vi "系统设置.vi"() -> ()   [LabVIEW 2016]
uses:
  <vilib>/Utility/miscctls.llb/LVPointTypeDef.ctl
  <vilib>/ptbypt/NI_PtbyPt.lvlib
  <vilib>/Utility/config.llb/NI_LVConfig.lvlib
  PLC/PLC.lvlib
panel:
  in  "模块启用配置":bool
  in  "短信报警设置":bool
  in  "首页显示设置":bool
  in  "跨度核查":bool
  in  "空白核查":bool
  out "选项卡控件":enum32{"自由设定", "国标协议", "流量设定"}(tab)
  in  "24H周期设置":bool[](xcontrol)
  in  "运行间隔":i16=4 min=1 max=24
  in  "流量阈值":dbl=4.0 min=1.0 max=24.0
  in  "时间阈值":u16=4 min=1 max=24
  in  "周期设置":enum16{"自由设定", "国标协议", "流量设定"}(ring)
  out "x = y?":bool
  in  "质控启动日期":string(combo)="关闭"
  in  "跨度核查时间":u16(ring)=6 items=["00H", "01H", "02H", "03H", "04H", "05H", "06H", "07H", "08H", "09H", "10H", "11H", "12H", "13H", "14H", "15H", "16H", "17H", "18H", "19H", "20H", "21H", "22H", "23H", "关闭"]
  in  "空白核查时间":u16(ring)=2 items=["00H", "01H", "02H", "03H", "04H", "05H", "06H", "07H", "08H", "09H", "10H", "11H", "12H", "13H", "14H", "15H", "16H", "17H", "18H", "19H", "20H", "21H", "22H", "23H", "关闭"]
  in  "CODCr":bool
  in  "总磷总氮":bool
  in  "氨氮":bool
  in  "CODmn":bool
  in  "多参数":bool
  in  "输入密码":dbl
  in  "布尔":bool
  in  "副屏显示设置":bool
  in  "开机启动":bool caption="氨氮禁用"
  in  "运行模式":enum16{"维护模式", "常规模式", "应急模式", "质控模式"}(ring)
  # "注：周期设置分为自由设定和国标协议两种。\n1：选择自由设定情况下：运行间隔将不可选用并变灰色，周期设置可自由手动勾选\n2：选择国标协议情况下：周期时间将由运行间隔选择的时间决定，下方周期设置被禁用并无法手动勾选。\n3：选择流量设定情况下：瞬时流量连续超过流量阈值到达时间阈值设定值，仪器将自动开启测量。"
  # "自动运行启动参数"
  # "质控频次："
  # "空白核查时间："
  # "跨度核查时间："
  # "启动周期设置"
  # "m3/S"
  # "秒"
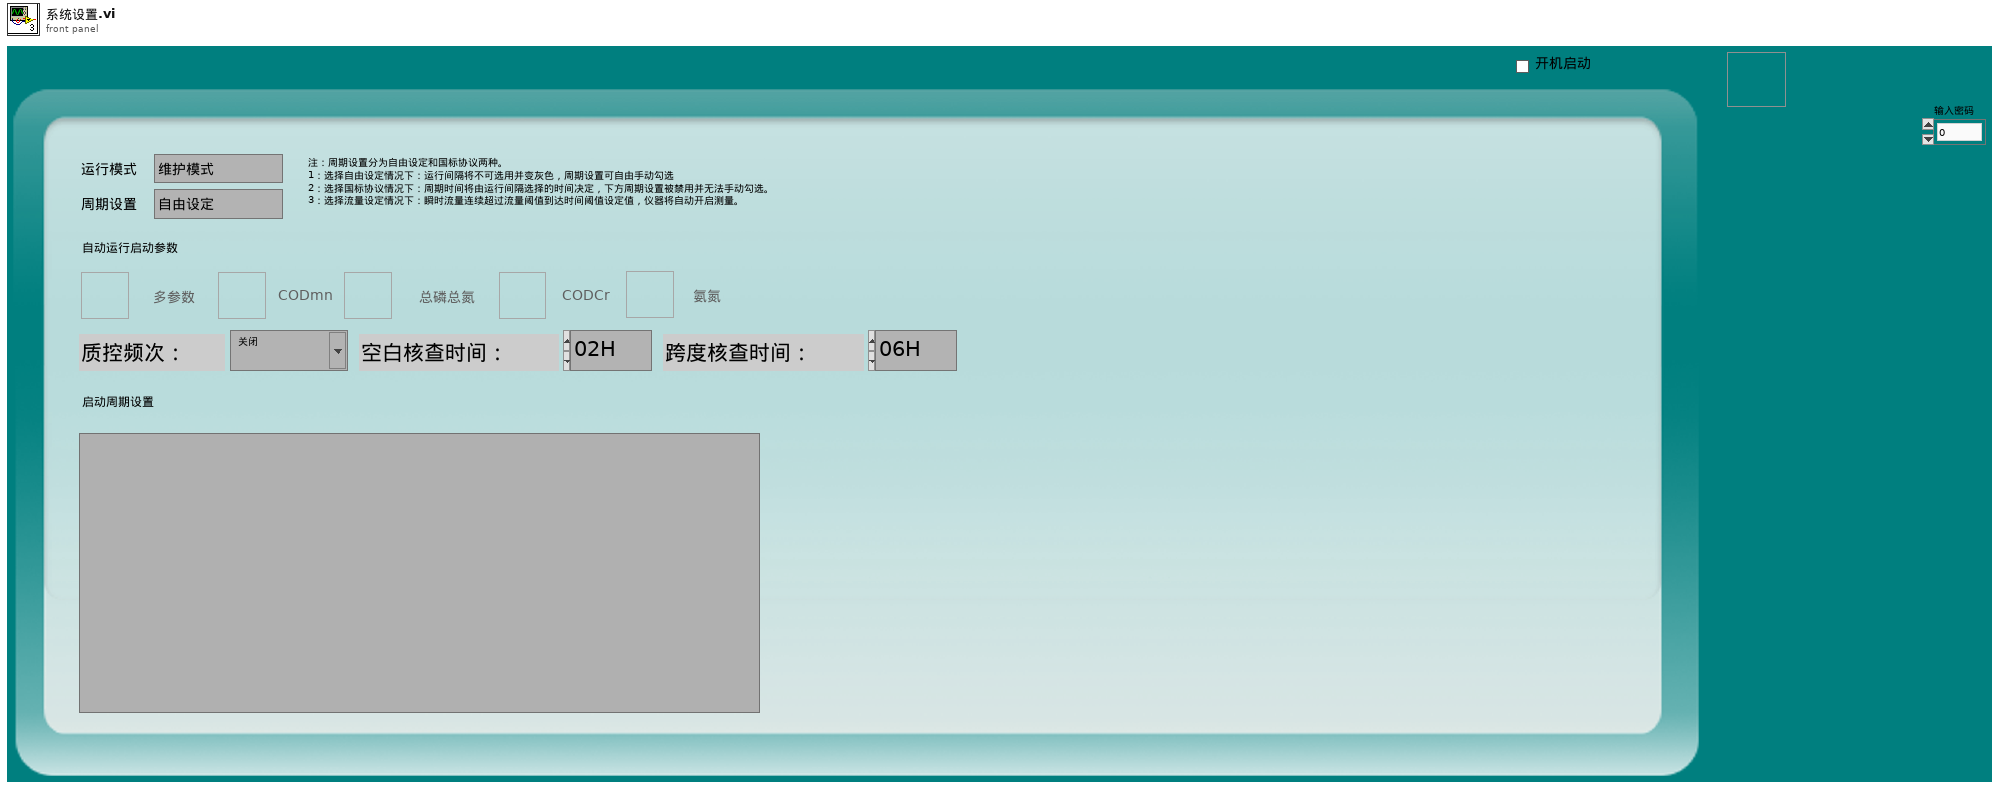
[diagram p1: front panel]
types:
  T1 = typedef "NI_LVConfig.lvlib/Config Data RefNum.ctl" = refnum<k1>
  T2 = typedef "LVPointTypeDef.ctl" = cluster{"Horizontal":i16, "Vertical":i16}
  T3 = enum8{"Enabled", "Disabled", "Disabled and Grayed Out"}
  T4 = enum32{"Bad", "Idle", "Run top level", "Running"}
  T5 = enum32{"Invalid", "Standard", "Closed", "Hidden", "Minimized", "Maximized"}
  T6 = cluster{"运行模式":enum16{"维护模式", "常规模式", "应急模式", "质控模式"}}
  T7 = cluster{"测量模式":enum16{"水样测量", "标样核查", "零点核查", "跨度核查", "空白测试", "加标回收", "平行样", "校零", "校标"}}
  T8 = cluster{"站号":u16, "量程切换":enum32{"H", "L", "AUTO"}, "控制命令":enum16{"启动测量", "标样核查", "零点核查", "跨度核查", "空白测试", "平行样测试", "加标回收", "空白校准", "标样校准", "初始化（清洗）", "停止测试", "仪器重启", "校时", "模式设置", "测量间隔设置"}, "模式设置":enum16{"待机", "连续模式", "周期模式", "定点模式", "受控模式", "手动模式"}, "测量间隔":u16}
  T9 = enum16{"启动测量", "标样核查", "零点核查", "跨度核查", "空白测试", "平行样测试", "加标回收", "空白校准", "标样校准", "初始化（清洗）", "停止测试", "仪器重启", "校时", "模式设置", "测量间隔设置"}
  T10 = cluster{"测试模式":enum16{"正常测试", "集成干预"}, "参数启用":cluster{"氨氮":bool, "总磷总氮":bool, "CODMn":bool, "CODcr":bool, "多参数":bool}}
  T11 = cluster{"运行模式":enum16{"维护模式", "常规模式", "应急模式", "质控模式"}, "质控频次":enum16{"关闭", "每天", "星期一", "星期二", "星期三", "星期四", "星期五", "星期六", "星期日"}, "空白核查时间":u16, "跨度核查时间":u16, "24H周期设置":bool[]}
  T12 = typedef "LVDateTimeRec.ctl" = cluster{"秒数的小数部分":dbl, "秒":i32, "分":i32, "时":i32, "日":i32, "月":i32, "年":i32, "天数（周）":i32, "天数（年）":i32, "DST":i32}
  T13 = cluster{"水样测试量程模式":enum16{"H", "L", "AUTO"}, "空白核查量程模式":enum16{"H", "L", "AUTO"}, "跨度核查量程模式":enum16{"H", "L", "AUTO"}}
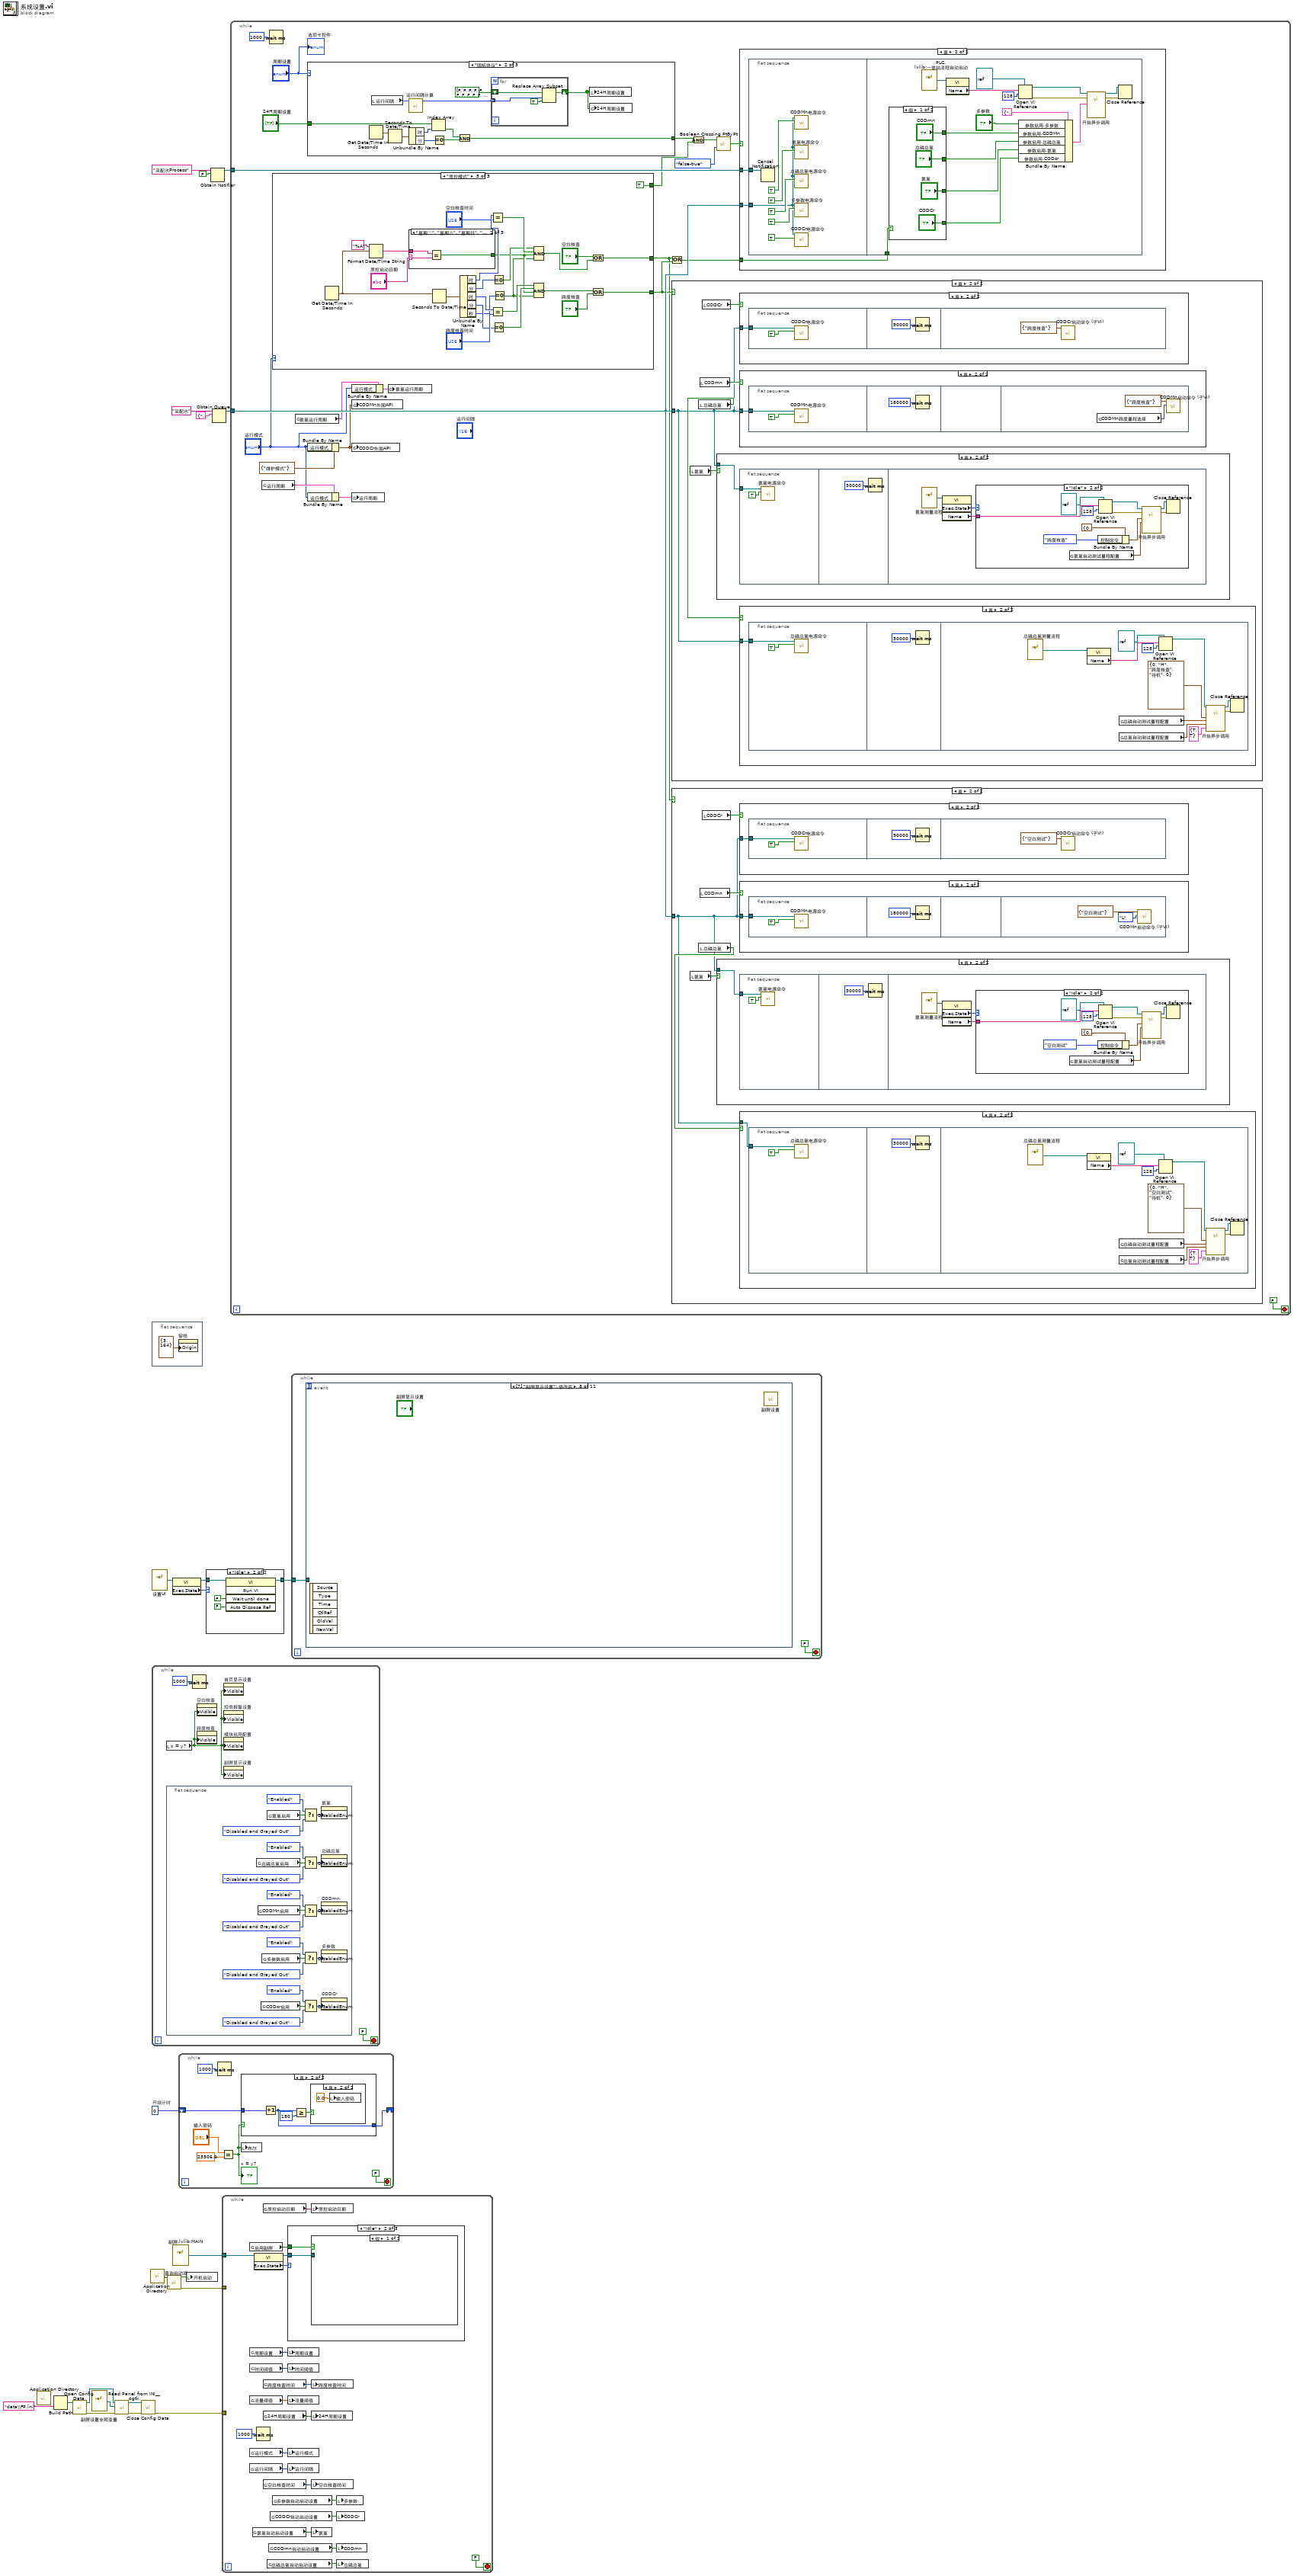
[diagram p0: block diagram]
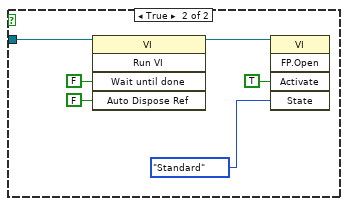
[diagram p6: hidden frame]
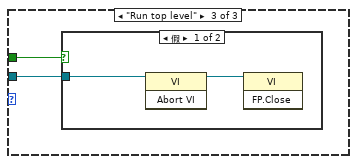
[diagram p7: hidden frame]
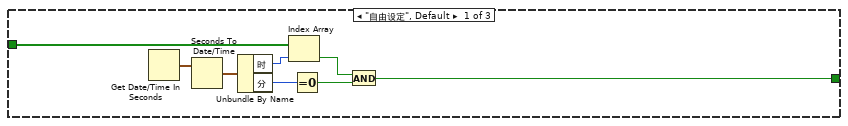
[diagram p9: hidden frame]
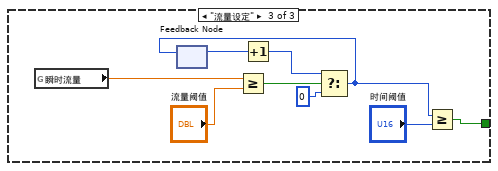
[diagram p10: hidden frame]
diagram:
  w18 = u32 0  # 开锁计时
  n1 = call <vilib>:"Application Directory.vi"() -> ()  [unwired: 1 out]
  n2 = Build Path(name or relative path="data\\FP.ini" ("名称或相对路径")) -> (appended path=w7:path)  [unwired: 1 in]
  n3 = call <vilib>:"Open Config Data.vi"("configuration file path"=w7) -> ("error out"=w6:errorcluster, "refnum"=w3:T1)  [unwired: 8 in, 1 out]
  n4 = vi-ref "副屏设置全局变量.vi"() -> (w4:refnum<vi>)
  n5 = call <userlib>:"Read Panel from INI__ogtk.vi"("error in (no error)"=w6, "VI ref"=w4, "refnum"=w3) -> ("error out"=w5:errorcluster, "refnum out"=w2:T1)  [unwired: 7 in]
  n6 = call <vilib>:"Close Config Data.vi"("error in (no error)"=w5, "refnum"=w2) -> ("error out"=w1:errorcluster)  [unwired: 8 in, 1 out]
  n7 = call <vilib>:"Application Directory.vi"() -> ("Application Directory"=w20:path)
  n8 = flat-sequence {
    frame #0 {
      n9 = property on="窗格" class="Pane"("Origin"=T2 {"Horizontal"=3, "Vertical"=164} ("原点")) -> ()  [unwired: 2 in, 2 out]
    }
  }
  n10 = vi-ref "设置UI.vi"() -> (w13:refnum<vi>)
  n11 = while {
    stop <- FALSE stop-if-true
    n12 = local read "x = y?"() -> (w25:bool)
    n13 = flat-sequence {
      frame #0 {
        n14 = global read "系统设置全局变量.vi" "总磷总氮启用"() -> (w35:bool)
        n15 = global read "系统设置全局变量.vi" "CODMn启用"() -> (w33:bool)
        n16 = global read "系统设置全局变量.vi" "CODcr启用"() -> (w34:bool)
        n17 = global read "系统设置全局变量.vi" "多参数启用"() -> (w32:bool)
        n18 = global read "系统设置全局变量.vi" "氨氮启用"() -> (w28:bool)
        n19 = Select(t=T3."Enabled" ("禁用"), s=w28, f=T3."Disabled and Grayed Out" ("禁用")) -> (s? t:f=w36:T3)
        n20 = Select(t=T3."Enabled" ("禁用"), s=w35, f=T3."Disabled and Grayed Out" ("禁用")) -> (s? t:f=w30:T3)
        n21 = Select(t=T3."Enabled" ("禁用"), s=w33, f=T3."Disabled and Grayed Out" ("禁用")) -> (s? t:f=w37:T3)
        n22 = Select(t=T3."Enabled" ("禁用"), s=w32, f=T3."Disabled and Grayed Out" ("禁用")) -> (s? t:f=w31:T3)
        n23 = Select(t=T3."Enabled" ("禁用"), s=w34, f=T3."Disabled and Grayed Out" ("禁用")) -> (s? t:f=w47:T3)
        n24 = property on="氨氮" class="Bool (严格)"("DisabledEnum"=w36) -> ()  [unwired: 2 in, 2 out]
        n25 = property on="总磷总氮" class="Bool (严格)"("DisabledEnum"=w30) -> ()  [unwired: 2 in, 2 out]
        n26 = property on="CODmn" class="Bool (严格)"("DisabledEnum"=w37) -> ()  [unwired: 2 in, 2 out]
        n27 = property on="多参数" class="Bool (严格)"("DisabledEnum"=w31) -> ()  [unwired: 2 in, 2 out]
        n28 = property on="CODCr" class="Bool (严格)"("DisabledEnum"=w47) -> ()  [unwired: 2 in, 2 out]
      }
    }
    n29 = Wait (ms)(milliseconds to wait=u32 1000 ("等待时间（毫秒）")) -> ()  [unwired: 1 out]
    n30 = property on="空白核查" class="Bool"("Visible"=w25) -> ()  [unwired: 2 in, 2 out]
    n31 = property on="跨度核查" class="Bool"("Visible"=w25) -> ()  [unwired: 2 in, 2 out]
    n32 = property on="首页显示设置" class="Bool"("Visible"=w25) -> ()  [unwired: 2 in, 2 out]
    n33 = property on="短信报警设置" class="Bool"("Visible"=w25) -> ()  [unwired: 2 in, 2 out]
    n34 = property on="模块启用配置" class="Bool"("Visible"=w25) -> ()  [unwired: 2 in, 2 out]
    n35 = property on="副屏显示设置" class="Bool"("Visible"=w25) -> ()  [unwired: 2 in, 2 out]
  }
  n36 = call "查询启动项.vi"("启动文件路径"=w20) -> ("error out"=w9:errorcluster, "包含启动项"=w19:bool)  [unwired: 9 in]
  n37 = property class="VI"(reference=w13) -> (reference out=w11:refnum<vi>, "Exec.State"=w12:T4)  [unwired: 1 in, 1 out]
  n38 = vi-ref "副屏.lvlib:MAIN.vi"() -> (w14:refnum<vi>)
  n39 = while {
    shift-right: [w49] -> _
    shift-left: w18 -> [w50]
    stop <- FALSE stop-if-true
    n40 = Wait (ms)(milliseconds to wait=u32 1000 ("等待时间（毫秒）")) -> ()  [unwired: 1 out]
    n41 = Equal?(x="输入密码", y=23506.0) -> (x = y?=w48:bool)
    "x = y?" <- w48
    n42 = case shown="真" w48 {
      tunnel: w50 -> [_ w58]
      tunnel: [_ w57] -> w49
      frame False {
      }
      frame True {
        n43 = Increment(x=w58) -> (x+1=w57:u32)
        n44 = Greater Or Equal?(x=w57, y=u32 180) -> (x >= y?=w55:bool)
        n45 = case shown="真" w55 {
          frame False {
          }
          frame True {
            n46 = local write "输入密码"(0.0 ("输入密码")) -> ()
          }
        }
      }
    }
    n47 = local write "布尔"(w48) -> ()
  }
  n48 = local write "开机启动"(w19) -> ()
  n49 = case shown="\"Idle\"" w12 {
    tunnel: w11 -> [w60 w64]
    tunnel: [w60 w63] -> w10
    frame "Bad", Default {
    }
    frame "Idle" {
      n50 = invoke class="VI" method="Run VI"(reference=w64, "Wait until done"=FALSE ("结束前等待"), "Auto Dispose Ref"=FALSE ("自动销毁引用")) -> (reference out=w63:refnum<vi>)  [unwired: 2 in, 4 out]
    }
  }
  n51 = Obtain Notifier(name (unnamed)="采配水Process" ("名称（未命名）"), notification data type=FALSE) -> (notifier out=w21:refnum<notifier>)  [unwired: 2 in, 2 out]
  n52 = Obtain Queue(name (unnamed)="采配水" ("名称（未命名）"), element data type=cluster{"命令":string, "数据":variant} {"命令"="", "数据"=variant}) -> (queue out=w15:refnum<queue>)  [unwired: 3 in, 2 out]
  n53 = while {
    tunnel: w14 -> [w76]
    tunnel: w9 -> [_]
    tunnel: w1 -> [_]
    stop <- FALSE stop-if-true
    n54 = global read "副屏设置全局变量.vi" "启用副屏"() -> (w74:bool)
    n55 = global read "系统设置全局变量.vi" "周期设置"() -> (w69:enum16{"自由设定", "国标协议", "流量设定"})
    n56 = global read "系统设置全局变量.vi" "时间阈值"() -> (w65:u16)
    n57 = global read "系统设置全局变量.vi" "流量阈值"() -> (w66:dbl)
    n58 = global read "系统设置全局变量.vi" "运行模式"() -> (w67:enum16{"维护模式", "常规模式", "应急模式", "质控模式"})
    n59 = global read "系统设置全局变量.vi" "运行间隔"() -> (w68:i16)
    n60 = global read "系统设置全局变量.vi" "氨氮自动启动设置"() -> (w81:bool)
    n61 = property class="VI"(reference=w76) -> (reference out=w73:refnum<vi>, "Exec.State"=w75:T4)  [unwired: 1 in, 1 out]
    n62 = Wait (ms)(milliseconds to wait=u32 1000 ("等待时间（毫秒）")) -> ()  [unwired: 1 out]
    n63 = global read "系统设置全局变量.vi" "质控启动日期"() -> (w72:string)
    n64 = global read "系统设置全局变量.vi" "跨度核查时间"() -> (w70:u16)
    n65 = global read "系统设置全局变量.vi" "24H周期设置"() -> (w82:bool[])
    n66 = global read "系统设置全局变量.vi" "空白核查时间"() -> (w71:u16)
    n67 = global read "系统设置全局变量.vi" "总磷总氮自动启动设置"() -> (w79:bool)
    n68 = global read "系统设置全局变量.vi" "CODmn自动启动设置"() -> (w78:bool)
    n69 = global read "系统设置全局变量.vi" "CODCr自动启动设置"() -> (w80:bool)
    n70 = global read "系统设置全局变量.vi" "多参数自动启动设置"() -> (w77:bool)
    n71 = case shown="\"Idle\"" w75 {
      tunnel: w74 -> [_ w85 w93]
      tunnel: w73 -> [_ w86 w94]
      frame "Bad", Default {
      }
      frame "Idle" {
        n72 = case shown="假" w85 {
          tunnel: w86 -> [_ w92]
          frame False {
          }
          frame True {
            n73 = invoke class="VI" method="Run VI"(reference=w92, "Wait until done"=FALSE ("结束前等待"), "Auto Dispose Ref"=FALSE ("自动销毁引用")) -> (reference out=w87:refnum<vi>)  [unwired: 2 in, 4 out]
            n74 = invoke class="VI" method="FP.Open"(reference=w87, "Activate"=TRUE ("激活？"), "State"=T5."Standard" ("状态")) -> ()  [unwired: 2 in, 5 out]
          }
        }
      }
      frame "Run top level" {
        n75 = case shown="假" w93 {
          tunnel: w94 -> [w95 _]
          frame False {
            n76 = invoke class="VI" method="Abort VI"(reference=w95) -> (reference out=w96:refnum<vi>)  [unwired: 2 in, 2 out]
            n77 = invoke class="VI" method="FP.Close"(reference=w96) -> ()  [unwired: 2 in, 3 out]
          }
          frame True {
          }
        }
      }
    }
    n78 = local write "周期设置"(w69) -> ()
    n79 = local write "时间阈值"(w65) -> ()
    n80 = local write "流量阈值"(w66) -> ()
    n81 = local write "运行模式"(w67) -> ()
    n82 = local write "运行间隔"(w68) -> ()
    n83 = local write "质控启动日期"(w72) -> ()
    n84 = local write "跨度核查时间"(w70) -> ()
    n85 = local write "24H周期设置"(w82) -> ()
    n86 = local write "空白核查时间"(w71) -> ()
    n87 = local write "氨氮"(w81) -> ()
    n88 = local write "多参数"(w77) -> ()
    n89 = local write "CODCr"(w80) -> ()
    n90 = local write "CODmn"(w78) -> ()
    n91 = local write "总磷总氮"(w79) -> ()
  }
  n92 = while {
    tunnel: w21 -> [w115]
    tunnel: w15 -> [w111]
    stop <- FALSE stop-if-true
    n93 = global read "总磷总氮断电保存全局变量.vi" "运行周期"() -> (w99:T11)
    n94 = Wait (ms)(milliseconds to wait=u32 1000 ("等待时间（毫秒）")) -> ()  [unwired: 1 out]
    n95 = case shown="\"质控模式\"" "运行模式" {
      tunnel: [_ _ w280] -> w104
      tunnel: [_ _ w284] -> w103
      tunnel: [_ TRUE TRUE] -> w108
      frame "维护模式", Default {
      }
      frame "常规模式" {
      }
      frame "质控模式" {
        n96 = Get Date/Time In Seconds() -> (seconds since 1Jan1904=w291:timestamp)
        n97 = Format Date/Time String(time format string (%c)="%A" ("时间格式字符串(%c)"), seconds (now)=w291) -> (date/time string=w289:string)  [unwired: 1 in]
        n98 = case shown="\"星期二\", \"星期六\", \"星期日\", \"星期三\", \"星期四\", \"星期五\", \"星期一\"" "质控启动日期" {
          selector: "质控启动日期" -> [w307 _ _]
          tunnel: [w306 TRUE FALSE] -> w292
          tunnel: w289 -> [w305 _ _]
          frame "星期二", "星期六", "星期日", "星期三", "星期四", "星期五", "星期一" {
            n99 = Equal?(x=w305, y=w307) -> (x = y?=w306:bool)
          }
          frame "每天" {
          }
          frame "关闭", Default {
          }
        }
        n100 = Seconds To Date/Time(time stamp (now)=w291) -> (date time rec=w304:T12)  [unwired: 1 in]
        n101 = Unbundle By Name(w304) -> ("时"=w303:i32, "分"=w301:i32, "时"=w297:i32, "分"=w296:i32, "秒"=w288:i32)
        n102 = Equal?(x=w303, y="空白核查时间") -> (x = y?=w300:bool)
        n103 = Equal?(x=w297, y="跨度核查时间") -> (x = y?=w295:bool)
        n104 = Equal To 0?(x=w301) -> (x = 0?=w299:bool)
        n105 = Equal To 0?(x=w296) -> (x = 0?=w294:bool)
        n106 = Equal To 0?(x=w288) -> (x = 0?=w287:bool)
        n107 = Compound Arithmetic op=AND ("复合运算")(w299, w300, w292, w287) -> (w285:bool)
        n108 = Compound Arithmetic op=AND ("复合运算")(w295, w294, w292, w287) -> (w282:bool)
        n109 = Or(x="空白核查", y=w285) -> (x .or. y?=w284:bool)
        n110 = Or(x=w282, y="跨度核查") -> (x .or. y?=w280:bool)
      }
    }
    n111 = global read "氨氮断电保存全局变量.vi" "氨氮运行周期"() -> (w101:T11)
    n112 = case shown="\"国标协议\"" "周期设置" {
      tunnel: [w119 w126 w142] -> w107
      tunnel: "24H周期设置" -> [w118 w127 _]
      frame "自由设定", Default {
        n113 = Get Date/Time In Seconds() -> (seconds since 1Jan1904=w120:timestamp)
        n114 = Seconds To Date/Time(time stamp (now)=w120) -> (date time rec=w121:T12)  [unwired: 1 in]
        n115 = Unbundle By Name(w121) -> ("时"=w124:i32, "分"=w122:i32)
        n116 = Index Array(array=w118, index=w124) -> (element=w125:bool)
        n117 = Equal To 0?(x=w122) -> (x = 0?=w123:bool)
        n118 = And(x=w125, y=w123) -> (x .and. y?=w119:bool)
      }
      frame "国标协议" {
        n119 = Get Date/Time In Seconds() -> (seconds since 1Jan1904=w128:timestamp)
        n120 = local read "运行间隔"() -> (w137:i16)
        n121 = Seconds To Date/Time(time stamp (now)=w128) -> (date time rec=w129:T12)  [unwired: 1 in]
        n122 = call "运行间隔计算.vi"("运行周期"=w137) -> ("数组"=w136:i32[])  [unwired: 10 in]
        n123 = Unbundle By Name(w129) -> ("时"=w132:i32, "分"=w130:i32)
        n124 = Index Array(array=w127, index=w132) -> (element=w133:bool)
        n125 = Equal To 0?(x=w130) -> (x = 0?=w131:bool)
        n126 = And(x=w133, y=w131) -> (x .and. y?=w126:bool)
        n127 = for {
          tunnel: w136 -> [w140] mode=indexing
          shift-right: [w138] -> w134
          shift-left: bool[] [FALSE, FALSE, FALSE, FALSE, FALSE, FALSE, FALSE, FALSE, FALSE, FALSE, FALSE, FALSE, FALSE, FALSE, FALSE, FALSE, FALSE, FALSE, FALSE, FALSE, FALSE, FALSE, FALSE, FALSE] ("24H周期设置") -> [w141]
          n128 = Replace Array Subset(array=w141, new element=TRUE ("新元素/子数组"), index=w140) -> (w138:bool[])
        }
        n129 = local write "24H周期设置"(w134) -> ()
        n130 = global write "系统设置全局变量.vi" "24H周期设置"(w134) -> ()
      }
      frame "流量设定" {
        n131 = global read "流量计全局变量.vi" "瞬时流量"() -> (w150:dbl)
        n132 = feedback #1() -> (w147:i16)  [unwired: 1 in]
        n133 = Greater Or Equal?(x=w150, y="流量阈值") -> (x >= y?=w145:bool)
        n134 = Increment(x=w147) -> (x+1=w146:i16)
        n135 = Select(t=w146, s=w145, f=i16 0) -> (s? t:f=w144:i16)
        n136 = feedback-in #1(w144) -> ()
        n137 = Greater Or Equal?(x=w144, y="时间阈值") -> (x >= y?=w142:bool)
      }
    }
    n138 = Bundle By Name(cluster=T6 {"运行模式"=enum."维护模式"} ("外围API"), "运行模式"="运行模式") -> (w105:T6)
    n139 = Bundle By Name(cluster=w99, "运行模式"="运行模式") -> (w98:T11)
    n140 = Bundle By Name(cluster=w101, "运行模式"="运行模式") -> (w100:T11)
    n141 = global write "CODMN外部API.vi" "CODMn外围API"(w105) -> ()
    n142 = global write "CODCr外部API.vi" "CODCr外围API"(w105) -> ()
    n143 = global write "总磷总氮断电保存全局变量.vi" "运行周期"(w98) -> ()
    n144 = global write "氨氮断电保存全局变量.vi" "氨氮运行周期"(w100) -> ()
    n145 = Or(x=w103, y=w104) -> (x .or. y?=w102:bool)
    n146 = case shown="真" w104 {
      tunnel: w111 -> [_ w151]
      frame False {
      }
      frame True {
        n147 = local read "氨氮"() -> (w155:bool)
        n148 = local read "总磷总氮"() -> (w154:bool)
        n149 = local read "CODmn"() -> (w153:bool)
        n150 = local read "CODCr"() -> (w152:bool)
        n151 = case shown="真" w155 {
          tunnel: w151 -> [_ w182]
          frame False {
          }
          frame True {
            n152 = flat-sequence {
              tunnel: w182 -> [w183]
              frame #0 {
                n153 = call "氨氮电源命令.vi"("通电/断电"=TRUE, "队列"=w183) -> ()  [unwired: 9 in, 1 out]
              }
              frame #1 {
                n154 = Wait (ms)(milliseconds to wait=u32 30000 ("等待时间（毫秒）")) -> ()  [unwired: 1 out]
              }
              frame #2 {
                n155 = vi-ref "氨氮测量流程.vi"() -> (w188:refnum<vi>)
                n156 = property class="VI"(reference=w188) -> ("Exec.State"=w186:T4, "Name"=w187:string)  [unwired: 1 in, 2 out]
                n157 = case shown="\"Idle\"" w186 {
                  tunnel: w187 -> [_ w196]
                  frame "Bad", Default {
                  }
                  frame "Idle" {
                    n158 = global read "氨氮断电保存全局变量.vi" "氨氮自动测试量程配置"() -> (w189:T13)
                    n159 = Bundle By Name(cluster=T8 {"站号"=0, "量程切换"=enum."H", "控制命令"=enum."启动测量", "模式设置"=enum."待机", "测量间隔"=0} ("参数"), "控制命令"=T9."跨度核查") -> (w191:T8)
                    n160 = Open VI Reference(type specifier VI Refnum (for type only)=refnum<vi> refnum, vi path=w196, options=128 ("选项")) -> (vi reference=w192:refnum<vi>, error out=w197:errorcluster)  [unwired: 3 in]
                    n161 = call-by-ref "开始异步调用"(reference=w192, error in=w197, "量程模式"=w189, "参数"=w191) -> (reference out=w198:refnum<vi>, error out=w199:errorcluster)  [unwired: 10 in]
                    n162 = Close Reference(reference=w198, error in (no error)=w199) -> ()  [unwired: 1 out]
                  }
                }
              }
            }
          }
        }
        n163 = case shown="真" w152 {
          tunnel: w151 -> [_ w156]
          frame False {
          }
          frame True {
            n164 = flat-sequence {
              tunnel: w156 -> [w157]
              frame #0 {
                n165 = call "CODCr电源命令.vi"("通电/断电"=TRUE, "队列"=w157) -> ()  [unwired: 9 in, 1 out]
              }
              frame #1 {
                n166 = Wait (ms)(milliseconds to wait=u32 90000 ("等待时间（毫秒）")) -> ()  [unwired: 1 out]
              }
              frame #2 {
                n167 = call "CODCr启动命令 (子VI).vi"("启动测量模式"=T7 {"测量模式"=enum."跨度核查"}) -> ()  [unwired: 11 in]
              }
            }
          }
        }
        n168 = case shown="真" w153 {
          tunnel: w151 -> [_ w161]
          frame False {
          }
          frame True {
            n169 = flat-sequence {
              tunnel: w161 -> [w162]
              frame #0 {
                n170 = call "CODMn电源命令.vi"("通电/断电"=TRUE, "队列"=w162) -> ()  [unwired: 9 in, 1 out]
              }
              frame #1 {
                n171 = Wait (ms)(milliseconds to wait=u32 180000 ("等待时间（毫秒）")) -> ()  [unwired: 1 out]
              }
              frame #2 {
              }
              frame #3 {
                n172 = global read "CODMn断电保存全局变量.vi" "CODMn跨度量程选择"() -> (w165:enum32{"H", "L", "AUTO"})
                n173 = call "CODMn启动命令 (子VI).vi"("CODMn量程切换"=w165, "启动测量模式"=T7 {"测量模式"=enum."跨度核查"}) -> ()  [unwired: 10 in]
              }
            }
          }
        }
        n174 = case shown="真" w154 {
          tunnel: w151 -> [_ w167]
          frame False {
          }
          frame True {
            n175 = flat-sequence {
              tunnel: w167 -> [w169]
              frame #0 {
                n176 = call "总磷总氮电源命令.vi"("通电/断电"=TRUE, "队列"=w169) -> ()  [unwired: 9 in, 1 out]
              }
              frame #1 {
                n177 = Wait (ms)(milliseconds to wait=u32 30000 ("等待时间（毫秒）")) -> ()  [unwired: 1 out]
              }
              frame #2 {
                n178 = vi-ref "总磷总氮测量流程.vi"() -> (w179:refnum<vi>)
                n179 = property class="VI"(reference=w179) -> ("Name"=w180:string)  [unwired: 1 in, 2 out]
                n180 = global read "总磷总氮断电保存全局变量.vi" "总磷自动测试量程配置"() -> (w173:T13)
                n181 = global read "总磷总氮断电保存全局变量.vi" "总氮自动测试量程配置"() -> (w172:T13)
                n182 = Open VI Reference(type specifier VI Refnum (for type only)=refnum<vi> refnum, vi path=w180, options=128 ("选项")) -> (vi reference=w178:refnum<vi>)  [unwired: 3 in, 1 out]
                n183 = call-by-ref "开始异步调用"(reference=w178, "启动参数"=cluster{"总磷":bool, "总氮":bool} {"总磷"=TRUE, "总氮"=TRUE}, "总氮量程模式"=w172, "总磷量程模式"=w173, "参数"=T8 {"站号"=0, "量程切换"=enum."H", "控制命令"=enum."跨度核查", "模式设置"=enum."待机", "测量间隔"=0}) -> (reference out=w177:refnum<vi>, error out=w176:errorcluster)  [unwired: 9 in]
                n184 = Close Reference(reference=w177, error in (no error)=w176) -> ()  [unwired: 1 out]
              }
            }
          }
        }
      }
    }
    n185 = case shown="真" w103 {
      tunnel: w111 -> [_ w200]
      frame False {
      }
      frame True {
        n186 = local read "氨氮"() -> (w204:bool)
        n187 = local read "总磷总氮"() -> (w203:bool)
        n188 = local read "CODmn"() -> (w202:bool)
        n189 = local read "CODCr"() -> (w201:bool)
        n190 = case shown="真" w204 {
          tunnel: w200 -> [_ w231]
          frame False {
          }
          frame True {
            n191 = flat-sequence {
              tunnel: w231 -> [w232]
              frame #0 {
                n192 = call "氨氮电源命令.vi"("通电/断电"=TRUE, "队列"=w232) -> ()  [unwired: 9 in, 1 out]
              }
              frame #1 {
                n193 = Wait (ms)(milliseconds to wait=u32 30000 ("等待时间（毫秒）")) -> ()  [unwired: 1 out]
              }
              frame #2 {
                n194 = vi-ref "氨氮测量流程.vi"() -> (w237:refnum<vi>)
                n195 = property class="VI"(reference=w237) -> ("Exec.State"=w235:T4, "Name"=w236:string)  [unwired: 1 in, 2 out]
                n196 = case shown="\"Idle\"" w235 {
                  tunnel: w236 -> [_ w245]
                  frame "Bad", Default {
                  }
                  frame "Idle" {
                    n197 = global read "氨氮断电保存全局变量.vi" "氨氮自动测试量程配置"() -> (w238:T13)
                    n198 = Bundle By Name(cluster=T8 {"站号"=0, "量程切换"=enum."H", "控制命令"=enum."启动测量", "模式设置"=enum."待机", "测量间隔"=0} ("参数"), "控制命令"=T9."空白测试") -> (w240:T8)
                    n199 = Open VI Reference(type specifier VI Refnum (for type only)=refnum<vi> refnum, vi path=w245, options=128 ("选项")) -> (vi reference=w241:refnum<vi>, error out=w246:errorcluster)  [unwired: 3 in]
                    n200 = call-by-ref "开始异步调用"(reference=w241, error in=w246, "量程模式"=w238, "参数"=w240) -> (reference out=w247:refnum<vi>, error out=w248:errorcluster)  [unwired: 10 in]
                    n201 = Close Reference(reference=w247, error in (no error)=w248) -> ()  [unwired: 1 out]
                  }
                }
              }
            }
          }
        }
        n202 = case shown="真" w201 {
          tunnel: w200 -> [_ w205]
          frame False {
          }
          frame True {
            n203 = flat-sequence {
              tunnel: w205 -> [w206]
              frame #0 {
                n204 = call "CODCr电源命令.vi"("通电/断电"=TRUE, "队列"=w206) -> ()  [unwired: 9 in, 1 out]
              }
              frame #1 {
                n205 = Wait (ms)(milliseconds to wait=u32 90000 ("等待时间（毫秒）")) -> ()  [unwired: 1 out]
              }
              frame #2 {
                n206 = call "CODCr启动命令 (子VI).vi"("启动测量模式"=T7 {"测量模式"=enum."空白测试"}) -> ()  [unwired: 11 in]
              }
            }
          }
        }
        n207 = case shown="真" w202 {
          tunnel: w200 -> [_ w210]
          frame False {
          }
          frame True {
            n208 = flat-sequence {
              tunnel: w210 -> [w211]
              frame #0 {
                n209 = call "CODMn电源命令.vi"("通电/断电"=TRUE, "队列"=w211) -> ()  [unwired: 9 in, 1 out]
              }
              frame #1 {
                n210 = Wait (ms)(milliseconds to wait=u32 180000 ("等待时间（毫秒）")) -> ()  [unwired: 1 out]
              }
              frame #2 {
              }
              frame #3 {
                n211 = call "CODMn启动命令 (子VI).vi"("CODMn量程切换"=enum32{"H", "L", "AUTO"}."L", "启动测量模式"=T7 {"测量模式"=enum."空白测试"}) -> ()  [unwired: 10 in]
              }
            }
          }
        }
        n212 = case shown="真" w203 {
          tunnel: w200 -> [_ w216]
          frame False {
          }
          frame True {
            n213 = flat-sequence {
              tunnel: w216 -> [w218]
              frame #0 {
                n214 = call "总磷总氮电源命令.vi"("通电/断电"=TRUE, "队列"=w218) -> ()  [unwired: 9 in, 1 out]
              }
              frame #1 {
                n215 = Wait (ms)(milliseconds to wait=u32 30000 ("等待时间（毫秒）")) -> ()  [unwired: 1 out]
              }
              frame #2 {
                n216 = vi-ref "总磷总氮测量流程.vi"() -> (w228:refnum<vi>)
                n217 = property class="VI"(reference=w228) -> ("Name"=w229:string)  [unwired: 1 in, 2 out]
                n218 = global read "总磷总氮断电保存全局变量.vi" "总磷自动测试量程配置"() -> (w222:T13)
                n219 = global read "总磷总氮断电保存全局变量.vi" "总氮自动测试量程配置"() -> (w221:T13)
                n220 = Open VI Reference(type specifier VI Refnum (for type only)=refnum<vi> refnum, vi path=w229, options=128 ("选项")) -> (vi reference=w227:refnum<vi>)  [unwired: 3 in, 1 out]
                n221 = call-by-ref "开始异步调用"(reference=w227, "启动参数"=cluster{"总磷":bool, "总氮":bool} {"总磷"=TRUE, "总氮"=TRUE}, "总氮量程模式"=w221, "总磷量程模式"=w222, "参数"=T8 {"站号"=0, "量程切换"=enum."H", "控制命令"=enum."空白测试", "模式设置"=enum."待机", "测量间隔"=0}) -> (reference out=w226:refnum<vi>, error out=w225:errorcluster)  [unwired: 9 in]
                n222 = Close Reference(reference=w226, error in (no error)=w225) -> ()  [unwired: 1 out]
              }
            }
          }
        }
      }
    }
    n223 = And(x=w107, y=w108) -> (x .and. y?=w106:bool)
    n224 = call <vilib>:"Boolean Crossing PtByPt.vi"("direction"=enum16{"either", "false-true", "true-false"}."false-true", "input"=w106) -> ("crossing"=w113:bool)  [unwired: 1 in]
    n225 = case shown="真" w113 {
      tunnel: w115 -> [_ w251]
      tunnel: w111 -> [_ w250]
      tunnel: w102 -> [_ w249]
      frame False {
      }
      frame True {
        n226 = flat-sequence {
          tunnel: w251 -> [w258]
          tunnel: w250 -> [w252]
          tunnel: w249 -> [w259]
          frame #0 {
            n227 = Cancel Notification(0:w258) -> ()  [unwired: 1 in, 3 out]
            n228 = call "CODMn电源命令.vi"("通电/断电"=TRUE, "队列"=w252) -> ()  [unwired: 9 in, 1 out]
            n229 = call "氨氮电源命令.vi"("通电/断电"=TRUE, "队列"=w252) -> ()  [unwired: 9 in, 1 out]
            n230 = call "总磷总氮电源命令.vi"("通电/断电"=TRUE, "队列"=w252) -> ()  [unwired: 9 in, 1 out]
            n231 = call "多参数电源命令.vi"("通电/断电"=TRUE, "队列"=w252) -> ()  [unwired: 9 in, 1 out]
            n232 = call "CODCr电源命令.vi"("通电/断电"=TRUE, "队列"=w252) -> ()  [unwired: 9 in, 1 out]
          }
          frame #1 {
            n233 = case shown="假" w259 {
              tunnel: ["CODmn" _] -> w273
              tunnel: ["总磷总氮" _] -> w272
              tunnel: ["CODCr" _] -> w271
              tunnel: ["氨氮" _] -> w270
              frame False {
              }
              frame True {
              }
            }
            n234 = vi-ref "PLC.lvlib:一体站流程自动启动.vi"() -> (w267:refnum<vi>)
            n235 = property class="VI"(reference=w267) -> ("Name"=w268:string)  [unwired: 1 in, 2 out]
            n236 = Bundle By Name(cluster=T10 {"测试模式"=enum."正常测试", "参数启用"={"氨氮"=FALSE, "总磷总氮"=FALSE, "CODMn"=FALSE, "CODcr"=FALSE, "多参数"=FALSE}} ("参数"), "参数启用.多参数"="多参数", "参数启用.CODMn"=w273, "参数启用.总磷总氮"=w272, "参数启用.氨氮"=w270, "参数启用.CODcr"=w271) -> (w260:T10)
            n237 = Open VI Reference(type specifier VI Refnum (for type only)=refnum<vi> refnum, vi path=w268, options=128 ("选项")) -> (vi reference=w266:refnum<vi>, error out=w265:errorcluster)  [unwired: 3 in]
            n238 = call-by-ref "开始异步调用"(reference=w266, error in=w265, "参数"=w260) -> (reference out=w264:refnum<vi>, error out=w263:errorcluster)  [unwired: 11 in]
            n239 = Close Reference(reference=w264, error in (no error)=w263) -> ()  [unwired: 1 out]
          }
        }
      }
    }
    "选项卡控件" <- "周期设置"
  }
  n240 = while {
    tunnel: w10 -> [w310]
    stop <- FALSE stop-if-true
    n241 = event shown="[7] \"副屏显示设置\": 值改变" {
      selector: _ -> [_ _ _ _ _ _ _ _ _ _ _]
      dyn-events: _ -> [_ _ _ _ _ _ _ _ _ _ _]
      timeout: _ -> [_ _ _ _ _ _ _ _ _ _ _]
      tunnel: w310 -> [_ _ _ _ _ _ _ _ _ w364 _]
      event Timeout {
        n242 = event-data() -> ()  [unwired: 1 in, 3 out]
      }
      event "模块启用配置": Value Change {
        n243 = event-data() -> ()  [unwired: 1 in, 6 out]
        n244 = call "模块启用配置框.vi"() -> ()  [unwired: 12 in]
      }
      event "24H周期设置", "运行模式", "多参数", "CODmn", "氨氮", "总磷总氮", "CODCr", "质控启动日期", "空白核查时间", "跨度核查时间", "运行间隔", "周期设置", "流量阈值", "时间阈值": Value Change {
        n245 = event-data() -> ()  [unwired: 1 in, 6 out]
        n246 = flat-sequence {
          frame #0 {
            n247 = local read "氨氮"() -> (w324:bool)
            n248 = local read "运行间隔"() -> (w315:i16)
            n249 = local read "流量阈值"() -> (w312:dbl)
            n250 = local read "总磷总氮"() -> (w322:bool)
            n251 = local read "周期设置"() -> (w314:enum16{"自由设定", "国标协议", "流量设定"})
            n252 = local read "时间阈值"() -> (w313:u16)
            n253 = local read "运行模式"() -> (w325:enum16{"维护模式", "常规模式", "应急模式", "质控模式"})
            n254 = local read "CODmn"() -> (w321:bool)
            n255 = local read "CODCr"() -> (w323:bool)
            n256 = local read "多参数"() -> (w320:bool)
            n257 = local read "空白核查时间"() -> (w317:u16)
            n258 = local read "质控启动日期"() -> (w318:string)
            n259 = local read "24H周期设置"() -> (w319:bool[])
            n260 = local read "跨度核查时间"() -> (w316:u16)
            n261 = global write "系统设置全局变量.vi" "氨氮自动启动设置"(w324) -> ()
            n262 = global write "系统设置全局变量.vi" "运行间隔"(w315) -> ()
            n263 = global write "系统设置全局变量.vi" "流量阈值"(w312) -> ()
            n264 = global write "系统设置全局变量.vi" "CODCr自动启动设置"(w323) -> ()
            n265 = global write "系统设置全局变量.vi" "总磷总氮自动启动设置"(w322) -> ()
            n266 = global write "系统设置全局变量.vi" "周期设置"(w314) -> ()
            n267 = global write "系统设置全局变量.vi" "CODmn自动启动设置"(w321) -> ()
            n268 = global write "系统设置全局变量.vi" "时间阈值"(w313) -> ()
            n269 = global write "系统设置全局变量.vi" "多参数自动启动设置"(w320) -> ()
            n270 = global write "系统设置全局变量.vi" "运行模式"(w325) -> ()
            n271 = global write "系统设置全局变量.vi" "空白核查时间"(w317) -> ()
            n272 = global write "系统设置全局变量.vi" "质控启动日期"(w318) -> ()
            n273 = global write "系统设置全局变量.vi" "24H周期设置"(w319) -> ()
            n274 = global write "系统设置全局变量.vi" "跨度核查时间"(w316) -> ()
          }
          frame #1 {
            n275 = call <vilib>:"Application Directory.vi"() -> ("Application Directory"=w339:path)
            n276 = Build Path(base path=w339, name or relative path="data\\sys.ini" ("名称或相对路径")) -> (appended path=w337:path)
            n277 = call <vilib>:"Open Config Data.vi"("configuration file path"=w337) -> ("error out"=w333:errorcluster, "refnum"=w336:T1)  [unwired: 8 in, 1 out]
            n278 = vi-ref "系统设置全局变量.vi"() -> (w335:refnum<vi>)
            n279 = call <userlib>:"Write Panel to INI__ogtk.vi"("error in (no error)"=w333, "VI ref"=w335, "refnum"=w336) -> ("error out"=w332:errorcluster, "refnum out"=w334:T1)  [unwired: 7 in]
            n280 = call <vilib>:"Close Config Data.vi"("error in (no error)"=w332, "refnum"=w334) -> ("error out"=w327:errorcluster, "file path"=w326:path)  [unwired: 8 in]
            n281 = Open/Create/Replace File(file path (use dialog)=w326, error in=w327) -> (refnum out=w330:refnum<file>, error out=w331:errorcluster)  [unwired: 4 in, 1 out]
            n282 = Flush File(refnum=w330, error in=w331) -> (refnum out=w329:refnum<file>, error out=w328:errorcluster)
            n283 = Close File(refnum=w329, error in=w328) -> ()  [unwired: 2 out]
          }
        }
      }
      event "运行间隔": Mouse Down {
        n284 = event-data() -> ("CtlRef"=w343:refnum<vi>)  [unwired: 1 in, 7 out]
        n285 = property class="DigNum (严格)"(reference=w343) -> (reference out=w342:refnum<vi>, "Value"=w341:i16)  [unwired: 1 in, 1 out]
        n286 = call "数字键盘.vi"("OldNumber"=w341) -> ("NewNumber"=w340:sgl)
        n287 = property class="DigNum (严格)"(reference=w342, "Val(Sgnl)"=w340) -> ()  [unwired: 1 in, 2 out]
      }
      event "流量阈值": Mouse Down {
        n288 = event-data() -> ("CtlRef"=w347:refnum<vi>)  [unwired: 1 in, 7 out]
        n289 = property class="DigNum (严格)"(reference=w347) -> (reference out=w346:refnum<vi>, "Value"=w345:dbl)  [unwired: 1 in, 1 out]
        n290 = call "数字键盘.vi"("OldNumber"=w345) -> ("NewNumber"=w344:sgl)
        n291 = property class="DigNum (严格)"(reference=w346, "Val(Sgnl)"=w344) -> ()  [unwired: 1 in, 2 out]
      }
      event "时间阈值": Mouse Down {
        n292 = event-data() -> ("CtlRef"=w351:refnum<vi>)  [unwired: 1 in, 7 out]
        n293 = property class="DigNum (严格)"(reference=w351) -> (reference out=w350:refnum<vi>, "Value"=w349:u16)  [unwired: 1 in, 1 out]
        n294 = call "数字键盘.vi"("OldNumber"=w349) -> ("NewNumber"=w348:sgl)
        n295 = property class="DigNum (严格)"(reference=w350, "Val(Sgnl)"=w348) -> ()  [unwired: 1 in, 2 out]
      }
      event "开机启动": Value Change {
        n296 = event-data() -> ("NewVal"=w353:bool)  [unwired: 1 in, 5 out]
        n297 = call <vilib>:"Application Directory.vi"() -> ("Application Directory"=w352:path)
        n298 = case shown="真" w353 {
          tunnel: w352 -> [w355 w359]
          frame False {
            n299 = call "删除启动项.vi"("启动文件路径"=w355) -> ("删除标记"=w354:bool)  [unwired: 9 in, 1 out]
            n300 = case shown="真" w354 {
              frame False {
                n301 = local write "开机启动"(TRUE ("开机启动")) -> ()
                n302 = One Button Dialog(message="启动项删除失败" ("消息")) -> ()  [unwired: 1 in, 1 out]
              }
              frame True {
              }
            }
          }
          frame True {
            n303 = call "添加启动项.vi"("启动文件路径"=w359) -> ("添加成功标记"=w358:bool)  [unwired: 9 in, 1 out]
            n304 = case shown="真" w358 {
              frame False {
                n305 = local write "开机启动"(FALSE ("开机启动")) -> ()
                n306 = One Button Dialog(message="启动项添加失败" ("消息")) -> ()  [unwired: 1 in, 1 out]
              }
              frame True {
              }
            }
          }
        }
      }
      event "副屏显示设置": Value Change {
        n307 = event-data() -> ()  [unwired: 1 in, 6 out]
        n308 = call "副屏设置.vi"() -> ()  [unwired: 12 in]
      }
      event "首页显示设置": Value Change {
        n309 = event-data() -> ()  [unwired: 1 in, 6 out]
        n310 = call "首页显示设置.vi"() -> ()  [unwired: 12 in]
      }
      event "短信报警设置": Value Change {
        n311 = event-data() -> ()  [unwired: 1 in, 6 out]
        n312 = invoke class="VI" method="FP.Open"(reference=w364, "Activate"=TRUE ("激活？"), "State"=T5."Standard" ("状态")) -> ()  [unwired: 2 in, 5 out]
      }
      event "布尔": Value Change {
        n313 = event-data() -> ("OldVal"=w366:bool)  [unwired: 1 in, 5 out]
        n314 = case shown="假" w366 {
          tunnel: [w367 _] -> w365
          frame False {
            n315 = call "数字密码键盘.vi"() -> ("NewNumber"=w367:sgl)  [unwired: 1 in]
          }
          frame True {
          }
        }
        n316 = local write "输入密码"(w365) -> ()
      }
    }
  }
